vi "cross product start.vi"(0 "Moment Arm":T2, 11 "Force":T3) -> (8 "Torque  Vector":T1)   [LabVIEW 2019]
doc: "This subvi does the crossproduct using the avectors of a force and a moment arm.\n\nJuan Gamez\nP3600"
uses:
  typedefs/force vector.ctl
  typedefs/moment arm vector.ctl
  P2 sol pw/typedefs/torque vector.ctl
panel:
  out "Nz":dbl
  out "Ny":dbl
  out "Nx":dbl
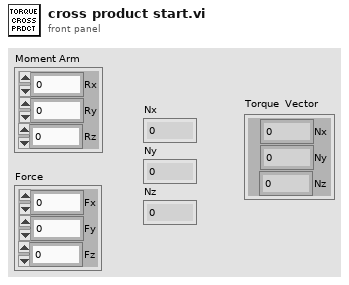
[diagram p1: front panel]
types:
  T1 = typedef "torque vector.ctl" = cluster{"Nx":dbl, "Ny":dbl, "Nz":dbl}
  T2 = typedef "moment arm vector.ctl" = cluster{"Rx":dbl, "Ry":dbl, "Rz":dbl}
  T3 = typedef "force vector.ctl" = cluster{"Fx":dbl, "Fy":dbl, "Fz":dbl}
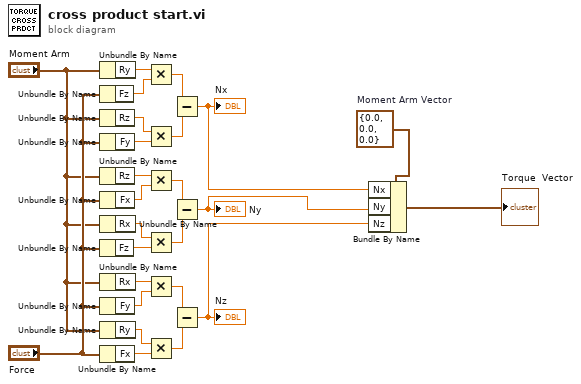
[diagram p0: block diagram]
diagram:
  w5 = T1 {"Nx"=0.0, "Ny"=0.0, "Nz"=0.0}  # Moment Arm Vector
  n1 = Unbundle By Name("Moment Arm") -> ("Ry"=w7:dbl)
  n2 = Unbundle By Name("Force") -> ("Fz"=w6:dbl)
  n3 = Unbundle By Name("Moment Arm") -> ("Rz"=w8:dbl)
  n4 = Unbundle By Name("Force") -> ("Fy"=w9:dbl)
  n5 = Unbundle By Name("Moment Arm") -> ("Rz"=w16:dbl)
  n6 = Unbundle By Name("Force") -> ("Fx"=w17:dbl)
  n7 = Unbundle By Name("Moment Arm") -> ("Rx"=w15:dbl)
  n8 = Unbundle By Name("Force") -> ("Fz"=w14:dbl)
  n9 = Unbundle By Name("Moment Arm") -> ("Rx"=w19:dbl)
  n10 = Unbundle By Name("Force") -> ("Fy"=w18:dbl)
  n11 = Unbundle By Name("Moment Arm") -> ("Ry"=w20:dbl)
  n12 = Unbundle By Name("Force") -> ("Fx"=w21:dbl)
  n13 = Multiply(x=w7, y=w6) -> (x*y=w10:dbl)
  n14 = Multiply(x=w8, y=w9) -> (x*y=w11:dbl)
  n15 = Multiply(x=w16, y=w17) -> (x*y=w13:dbl)
  n16 = Multiply(x=w15, y=w14) -> (x*y=w12:dbl)
  n17 = Multiply(x=w19, y=w18) -> (x*y=w22:dbl)
  n18 = Multiply(x=w20, y=w21) -> (x*y=w23:dbl)
  n19 = Subtract(x=w10, y=w11) -> (x-y=w4:dbl)
  "Nx" <- w4
  n20 = Subtract(x=w13, y=w12) -> (x-y=w3:dbl)
  "Ny" <- w3
  n21 = Subtract(x=w22, y=w23) -> (x-y=w2:dbl)
  "Nz" <- w2
  n22 = Bundle By Name(cluster=w5, "Nx"=w4, "Ny"=w3, "Nz"=w2) -> (→"Torque  Vector":T1)
